vi "Measure IV curves sequence in same file 6430.vi"() -> ()   [LabVIEW 2014]
uses:
  Environmental Chamber LabVIEW and Instruments/Drivers and Software/keithley_6430/Keithley 6430/Public/Data/Read (Single Point).vi
  <vilib>/Utility/file.llb/Write To Spreadsheet File (string).vi
  Environmental Chamber LabVIEW and Instruments/Drivers and Software/keithley_6430/Keithley 6430/Keithley 6430.lvlib
panel:
  in  "voltage settings":T1={"Vi (V)"=0.0, "Vf (V)"=0.3, "steps"=30.0, "# of curves"=1, "Delay (min)"=0.05} {"Delay (min)" min=0.0 format="%#_13g"; "# of curves" step=1}
  out "File path":path
  in  "STOP":bool
  out "2420 IV curve":cluster{"X":dbl[], "Y":dbl[]}[](graph)
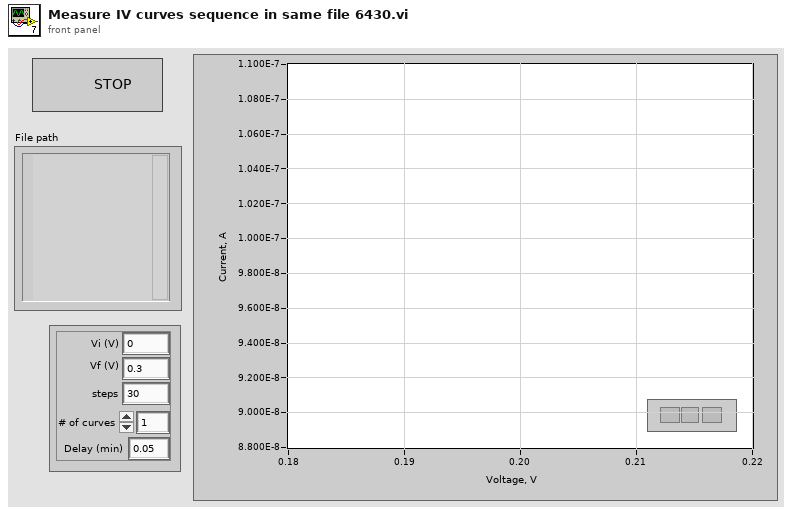
[diagram p1: front panel]
types:
  T1 = cluster{"Vi (V)":dbl, "Vf (V)":dbl, "steps":dbl, "# of curves":u32, "Delay (min)":dbl}
  T2 = enum16{"open", "open or create", "create or replace", "create", "open (read only)"}
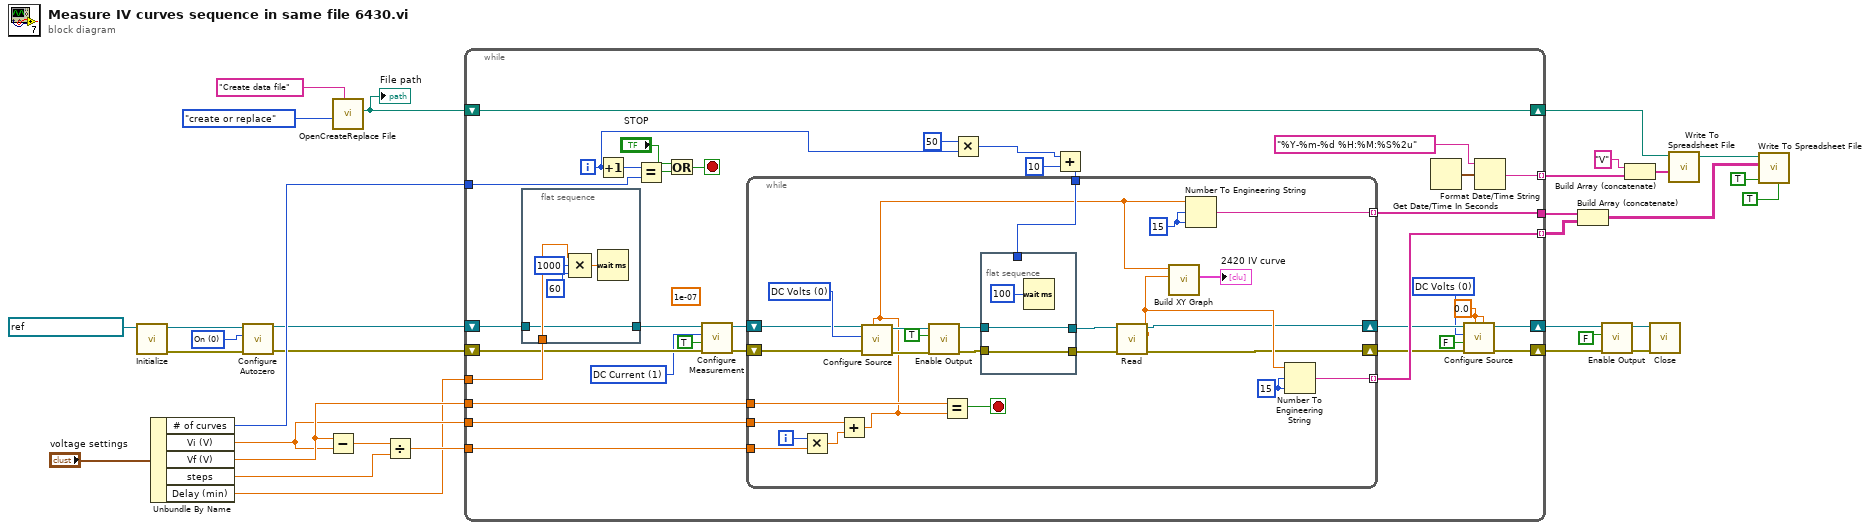
[diagram p0: block diagram]
diagram:
  w11 = u16 0 items=["On", "Off", "Once"] ("Autozero  (0: On)")
  n1 = call "Initialize.vi"("VISA resource name"=refnum<visa-resource-name> "GPIB2::19::INSTR") -> ("error out"=w10:errorcluster, "VISA resource name out"=w9:refnum<visa-resource-name>)  [unwired: 4 in, 5 out]
  n2 = Unbundle By Name("voltage settings") -> ("# of curves"=w26:u32, "Vi (V)"=w27:dbl, "Vf (V)"=w28:dbl, "steps"=w29:dbl, "Delay (min)"=w25:dbl)
  n3 = call "Configure Autozero.vi"("error in (no error)"=w10, "Autozero  (0: On)"=w11, "VISA resource name"=w9) -> ("error out"=w1:errorcluster, "VISA resource name out"=w2:refnum<visa-resource-name>)  [unwired: 7 in]
  n4 = Subtract(x=w28, y=w27) -> (x-y=w32:dbl)
  n5 = call "OpenCreateReplace File.vi"("prompt"="Create data file", "function (open:0)"=T2."create or replace") -> ("new file path"=w22:path)  [unwired: 6 in, 3 out]
  "File path" <- w22
  n6 = Divide(x=w32, y=w29) -> (x/y=w31:dbl)
  n7 = while {
    tunnel: w28 -> [w66]
    tunnel: w27 -> [w65]
    tunnel: w31 -> [w64]
    shift-right: [w43] -> w3
    shift-left: w1 -> [w36]
    shift-right: [w45] -> w4
    shift-left: w2 -> [w39]
    shift-right: [w57] -> w20
    shift-left: w22 -> [w57]
    tunnel: w26 -> [w59]
    tunnel: w25 -> [w58]
    tunnel: [w54] -> w17 mode=indexing
    tunnel: [w53] -> w15
    tunnel: [w52] -> w14 mode=indexing
    i -> [w51]
    stop <- w63 stop-if-true
    (unwired) 1e-07 ("Current Compliance [A]")
    w34 = u16 1 items=["DC Volts", "DC Current"] ("Measure Function (1: DC Current)")
    w40 = 0.0 ("V-Source Level [V]")
    w42 = u16 0 items=["DC Volts", "DC Current"] ("Source Function (0: DC Volts)")
    n8 = flat-sequence {
      tunnel: w39 -> [w67]
      tunnel: w58 -> [w68]
      tunnel: [w67] -> w38
      frame #0 {
        n9 = Compound Arithmetic op=MULTIPLY(w68, u32 1000 ("value"), u32 60 ("value")) -> (w71:dbl)
        n10 = Wait (ms)(milliseconds to wait=w71) -> ()  [unwired: 1 out]
      }
    }
    n11 = Increment(x=w51) -> (x+1=w61:i32)
    n12 = Equal?(x=w61, y=w59) -> (x = y?=w60:bool)
    n13 = Or(x="STOP", y=w60) -> (x .or. y?=w63:bool)
    n14 = call "Configure Measurement.vi"("error in (no error)"=w36, "Auto Range (T:Enable)"=TRUE, "Measure Function (1: DC Current)"=w34, "VISA resource name"=w38) -> ("error out"=w35:errorcluster, "VISA resource name out"=w37:refnum<visa-resource-name>)  [unwired: 6 in]
    n15 = Multiply(x=50, y=w51) -> (x*y=w49:i32)
    n16 = Add(x=w49, y=10) -> (x+y=w47:i32)
    n17 = while {
      tunnel: [w97] -> w52 mode=indexing
      shift-right: [w77] -> w44
      shift-left: w35 -> [w75]
      shift-right: [w79] -> w46
      shift-left: w37 -> [w76]
      tunnel: w64 -> [w87]
      tunnel: w65 -> [w96]
      tunnel: [w95] -> w53 mode=indexing
      tunnel: w66 -> [w89]
      tunnel: w47 -> [w86]
      i -> [w88]
      stop <- w90 stop-if-true
      w83 = u16 0 items=["DC Volts", "DC Current"] ("Source Function (0: DC Volts)")
      w92 = i16 15 ("precision (6)")
      w93 = i16 15 ("precision (6)")
      n18 = Multiply(x=w88, y=w87) -> (x*y=w94:dbl)
      n19 = Add(x=w96, y=w94) -> (x+y=w72:dbl)
      n20 = call "Configure Source.vi"("V-Source Level [V]"=w72, "error in (no error)"=w75, "Source Function (0: DC Volts)"=w83, "VISA resource name"=w76) -> ("error out"=w85:errorcluster, "VISA resource name out"=w84:refnum<visa-resource-name>)  [unwired: 6 in]
      n21 = call "Enable Output.vi"("error in (no error)"=w85, "Enable Output (F:Off)"=TRUE, "VISA resource name"=w84) -> ("error out"=w74:errorcluster, "VISA resource name out"=w73:refnum<visa-resource-name>)  [unwired: 7 in]
      n22 = Equal?(x=w89, y=w72) -> (x = y?=w90:bool)
      n23 = flat-sequence {
        tunnel: [w100] -> w80
        tunnel: w73 -> [w100]
        tunnel: w74 -> [w99]
        tunnel: [w99] -> w78
        tunnel: w86 -> [_]
        frame #0 {
          n24 = Wait (ms)(milliseconds to wait=100 ("x")) -> ()  [unwired: 1 out]
        }
      }
      n25 = call-poly "Read.vi"("error in (no error)"=w78, "VISA resource name"=w80) -> ("error out"=w77:errorcluster, "Measurement"=w81:dbl, "VISA resource name out"=w79:refnum<visa-resource-name>)  [unwired: 7 in]
      n26 = call "Build XY Graph"("Y Input"=w81, "X Input"=w72) -> ("XY Graph"=→"2420 IV curve":cluster{"X":dbl[], "Y":dbl[]}[])  [unwired: 8 in, 1 out]
      n27 = Number To Engineering String(2:w92, 3:w92, 4:w72) -> (0:w95:string)  [unwired: 1 in]
      n28 = Number To Engineering String(2:w93, 3:w93, 4:w81) -> (0:w97:string)  [unwired: 1 in]
    }
    n29 = Get Date/Time In Seconds() -> (seconds since 1Jan1904=w56:timestamp)
    n30 = call "Configure Source.vi"("I-Source Level [A]"=w40, "V-Source Level [V]"=w40, "error in (no error)"=w44, "Auto Range (T:Enable)"=FALSE, "Source Function (0: DC Volts)"=w42, "VISA resource name"=w46) -> ("error out"=w43:errorcluster, "VISA resource name out"=w45:refnum<visa-resource-name>)  [unwired: 4 in]
    n31 = Format Date/Time String(time format string (%c)="%Y-%m-%d %H:%M:%S%2u", seconds (now)=w56) -> (date/time string=w54:string)  [unwired: 1 in]
  }
  n32 = Build Array (concatenate)(w15, w14) -> (w13:string[][])
  n33 = call "Enable Output.vi"("error in (no error)"=w3, "Enable Output (F:Off)"=FALSE ("Output (F:Off)"), "VISA resource name"=w4) -> ("error out"=w5:errorcluster, "VISA resource name out"=w6:refnum<visa-resource-name>)  [unwired: 7 out]
  n34 = Build Array (concatenate)("V", w17) -> (w16:string[])
  n35 = call "Close.vi"("error in (no error)"=w5, "VISA resource name"=w6) -> ()  [unwired: 10 out]
  n36 = call-poly <vilib>:"Write To Spreadsheet File.vi"("1D data"=w16, "file path (dialog if empty)"=w20) -> ("new file path (Not A Path if cancelled)"=w19:path)  [unwired: 6 in]
  n37 = call-poly <vilib>:"Write To Spreadsheet File.vi"("transpose? (no:F)"=TRUE, "append to file? (new file:F)"=TRUE ("transpose? (no:F)"), "2D data"=w13, "file path (dialog if empty)"=w19) -> ()  [unwired: 4 in, 1 out]
